vi "Graficacion (SubVI).vi"(6 "Punto final de la onda":i32=2500 min=0 max=2500 step=1, 7 "Estados de los canales":T1, 8 "error in (no error)":errorcluster, 9 "Punto inicial de la onda":i32 min=0 max=2500 step=1, 10 "Mayor Precisión":bool, 11 "VISA Refnum in":refnum<visa-resource-name>) -> (0 "error out":errorcluster, 1 "Array":string[](array[string]), 2 "Gráfica":waveform(dbl)[](graph), 3 "VISA Refnum out":refnum<visa-resource-name>)   [LabVIEW 2014]
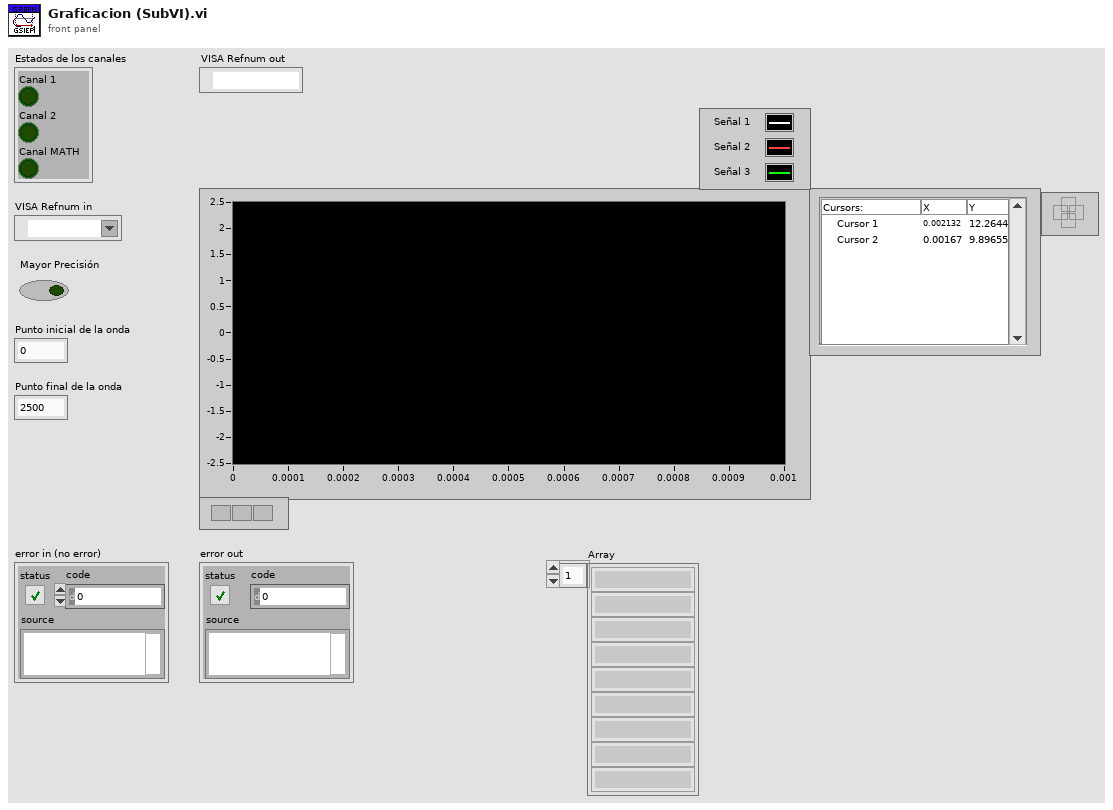
[diagram p1: front panel]
types:
  T1 = cluster{"Canal 1":bool, "Canal 2":bool, "Canal MATH":bool}
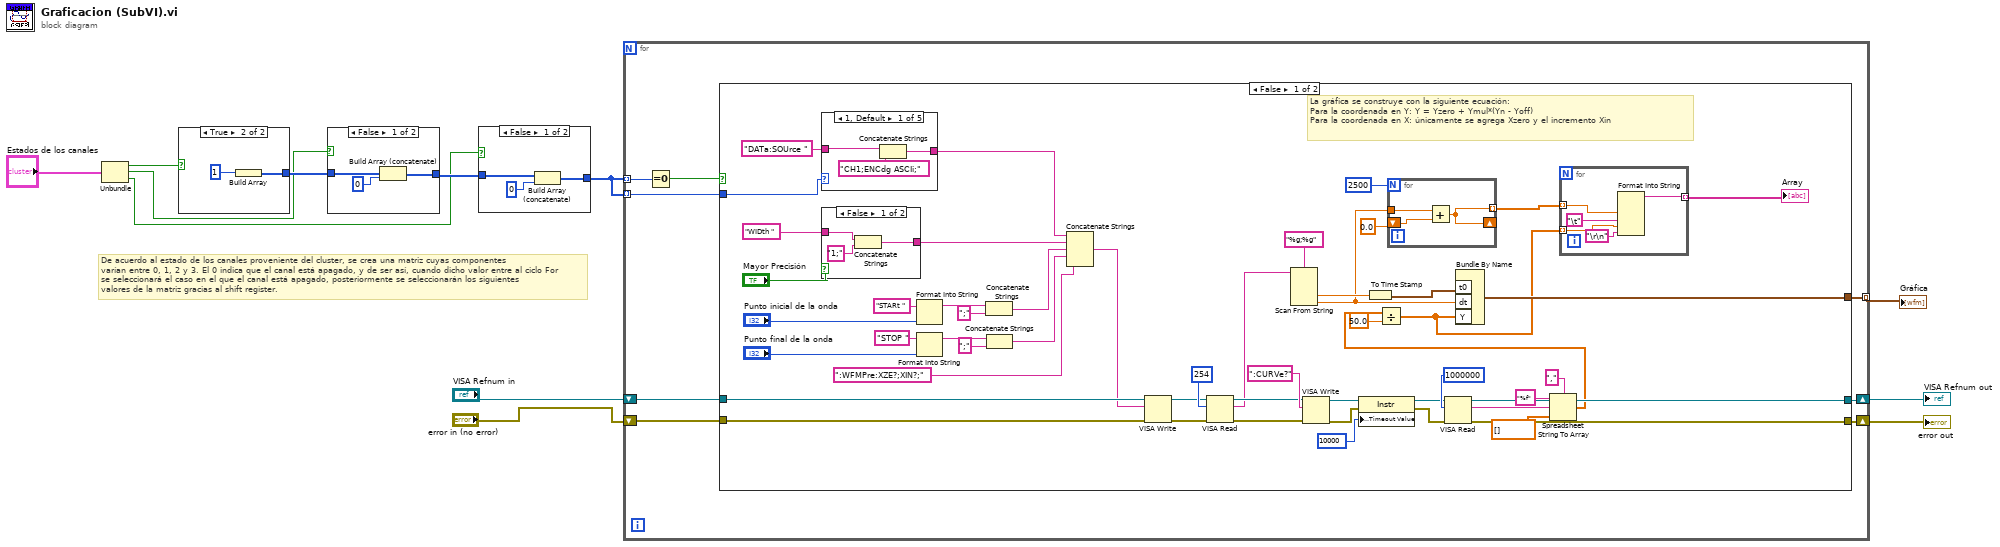
[diagram p0: block diagram]
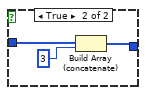
[diagram p2: hidden frame]
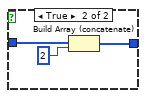
[diagram p3: hidden frame]
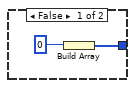
[diagram p4: hidden frame]
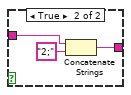
[diagram p5: hidden frame]
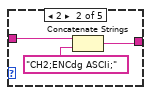
[diagram p6: hidden frame]
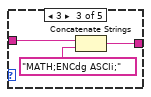
[diagram p7: hidden frame]
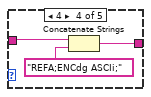
[diagram p8: hidden frame]
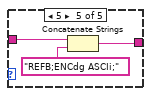
[diagram p9: hidden frame]
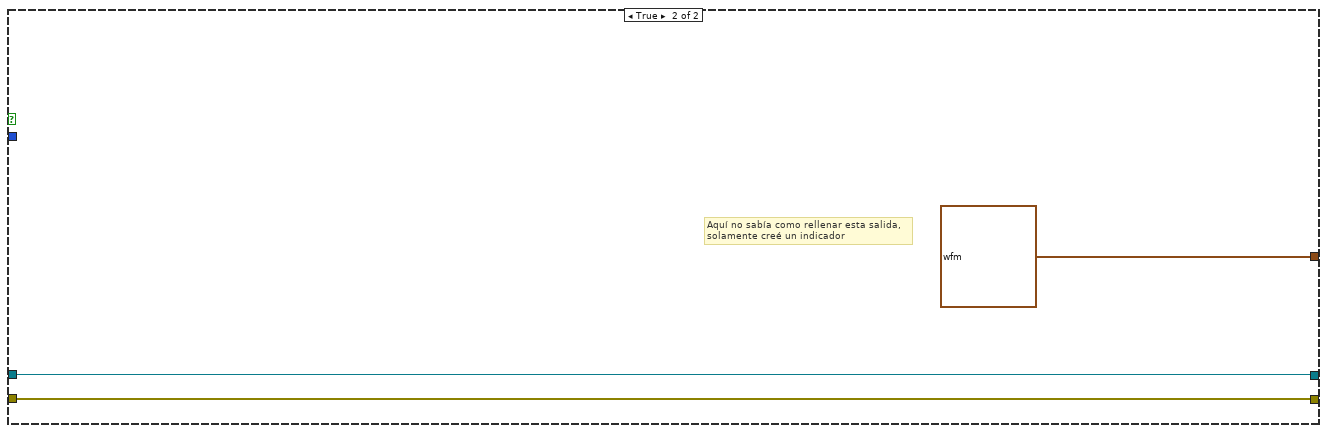
[diagram p10: hidden frame]
diagram:
  # "De acuerdo al estado de los canales proveniente del cluster, se crea una matriz cuyas componentes\nvarían entre 0, 1, 2 y 3. El 0 indica que el canal está apagado, y de ser así, cuando dicho valor entre al ciclo For\nse seleccionará el caso en el que el canal está apagado, posteriormente se seleccionarán los siguientes \nvalores de la matriz gracias al shift register."
  n1 = Unbundle("Estados de los canales") -> ("Canal 1"=w6:bool, "Canal 2"=w7:bool, "Canal MATH"=w8:bool)
  n2 = case shown="True" w6 {
    tunnel: [w13 w15] -> w9
    frame False {
      n3 = Build Array(0) -> (w13:i32[])
    }
    frame True {
      n4 = Build Array(1) -> (w15:i32[])
    }
  }
  n5 = case shown="False" w7 {
    tunnel: w9 -> [w19 w21]
    tunnel: [w17 w20] -> w10
    frame False {
      n6 = Build Array (concatenate)(w19, 0) -> (w17:i32[])
    }
    frame True {
      n7 = Build Array (concatenate)(w21, 2) -> (w20:i32[])
    }
  }
  n8 = case shown="False" w8 {
    tunnel: w10 -> [w25 w27]
    tunnel: [w23 w26] -> w11
    frame False {
      n9 = Build Array (concatenate)(w25, 0) -> (w23:i32[])
    }
    frame True {
      n10 = Build Array (concatenate)(w27, 3) -> (w26:i32[])
    }
  }
  n11 = for {
    tunnel: w11 -> [w31] mode=indexing
    shift-right: [w34] -> w3
    shift-left: "VISA Refnum in" -> [w36]
    shift-right: [w33] -> w4
    shift-left: "error in (no error)" -> [w35]
    tunnel: [w32] -> w5 mode=indexing
    tunnel: w11 -> [w30] mode=indexing
    n12 = Equal To 0?(x=w31) -> (x = 0?=w29:bool)
    n13 = case shown="False" w29 {
      tunnel: w36 -> [w87 w119]
      tunnel: w35 -> [w86 w118]
      tunnel: [w85 w119] -> w34
      tunnel: [w84 w118] -> w33
      tunnel: [w46 waveform(dbl) {"t0"=timestamp(0 s since 1904-01-01), "dt"=1.0, "Y"=[]}] -> w32
      tunnel: w30 -> [w48 _]
      frame False {
        # "La gráfica se construye con la siguiente ecuación:\nPara la coordenada en Y: Y = Yzero + Ymul*(Yn - Yoff)\nPara la coordenada en X: únicamente se agrega Xzero y el incremento Xin"
        n14 = case shown="1, Default" w48 {
          tunnel: "DATa:SOUrce " -> [w103 w107 w110 w111 w115]
          tunnel: [w102 w105 w108 w113 w114] -> w49
          frame 1, Default {
            n15 = Concatenate Strings(w103, "CH1;ENCdg ASCIi;") -> (w102:string)
          }
          frame 2 {
            n16 = Concatenate Strings(w107, "CH2;ENCdg ASCIi;") -> (w105:string)
          }
          frame 3 {
            n17 = Concatenate Strings(w110, "MATH;ENCdg ASCIi;") -> (w108:string)
          }
          frame 4 {
            n18 = Concatenate Strings(w111, "REFA;ENCdg ASCIi;") -> (w113:string)
          }
          frame 5 {
            n19 = Concatenate Strings(w115, "REFB;ENCdg ASCIi;") -> (w114:string)
          }
        }
        n20 = case shown="False" "Mayor Precisión" {
          tunnel: "WIDth " -> [w97 w100]
          tunnel: [w96 w99] -> w76
          frame False {
            n21 = Concatenate Strings(w97, "1;" ("string")) -> (w96:string)
          }
          frame True {
            n22 = Concatenate Strings(w100, "2;" ("string")) -> (w99:string)
          }
        }
        n23 = Format Into String(initial string="STARt ", "Punto inicial de la onda") -> (resulting string=w73:string)  [unwired: 2 in, 1 out]
        n24 = Format Into String(initial string="STOP ", "Punto final de la onda") -> (resulting string=w70:string)  [unwired: 2 in, 1 out]
        n25 = Concatenate Strings(w73, ";" ("string")) -> (w69:string)
        n26 = Concatenate Strings(w70, ";" ("string")) -> (w68:string)
        n27 = Concatenate Strings(w49, w76, w69, w68, ":WFMPre:XZE?;XIN?;") -> (w75:string)
        n28 = VISA Write(VISA resource name=w87, write buffer=w75, error in (no error)=w86) -> (VISA resource name out=w65:refnum<visa-resource-name>, error out=w64:errorcluster)  [unwired: 1 out]
        n29 = VISA Read(VISA resource name=w65, byte count=u32 254, error in (no error)=w64) -> (VISA resource name out=w63:refnum<visa-resource-name>, read buffer=w50:string, error out=w62:errorcluster)  [unwired: 1 out]
        n30 = Scan From String(format string="%g;%g", input string=w50) -> (output 1=w43:dbl, output 2=w41:dbl)  [unwired: 2 in, 5 out]
        n31 = VISA Write(VISA resource name=w63, write buffer=":CURVe?", error in (no error)=w62) -> (VISA resource name out=w59:refnum<visa-resource-name>, error out=w58:errorcluster)  [unwired: 1 out]
        n32 = property class="Instr"(reference=w59, error in=w58, "General Settings:Timeout Value"=u32 10000) -> (reference out=w57:refnum<visa-resource-name>, error out=w56:errorcluster)
        n33 = To Time Stamp(1:w43) -> (0:w45:timestamp)
        n34 = for {
          N: 2500 -> [_]
          tunnel: [w89] -> w39 mode=indexing
          tunnel: w41 -> [w90]
          shift-right: [w89] -> _
          shift-left: 0.0 -> [w88]
          n35 = Add(x=w90, y=w88) -> (x+y=w89:dbl)
        }
        n36 = VISA Read(VISA resource name=w57, byte count=u32 1000000, error in (no error)=w56) -> (VISA resource name out=w85:refnum<visa-resource-name>, read buffer=w52:string, error out=w84:errorcluster)  [unwired: 1 out]
        n37 = Spreadsheet String To Array(delimiter (Tab)=",", format string="%f", spreadsheet string=w52, array type (2D Dbl)=dbl[] []) -> (array=w44:dbl[])
        n38 = Divide(x=w44, y=50.0) -> (x/y=w42:dbl[])
        n39 = Bundle By Name("t0"=w45, "dt"=w41, "Y"=w42) -> (w46:waveform(dbl))  [unwired: 1 out]
        n40 = for {
          tunnel: [w95] -> w40 mode=indexing
          tunnel: w42 -> [w92] mode=indexing
          tunnel: w39 -> [w91] mode=indexing
          n41 = Format Into String(w91, "\t", w92, "\r\n") -> (resulting string=w95:string)  [unwired: 3 in, 1 out]
        }
        "Array" <- w40
      }
      frame True {
        # "Aquí no sabía como rellenar esta salida,\nsolamente creé un indicador"
      }
    }
  }
  "VISA Refnum out" <- w3
  "error out" <- w4
  "Gráfica" <- w5
